vi "Find API Tester Path.vi"(8 "error in":errorcluster, 11 "DQMH Library Ref":refnum<vi>) -> (0 "error out":errorcluster, 2 "Api tester found?":bool, 3 "API Tester Path":path)   [LabVIEW 2020, in "Panther Dashboard.lvlib"]
uses:
  Panther Dashboard.lvlib
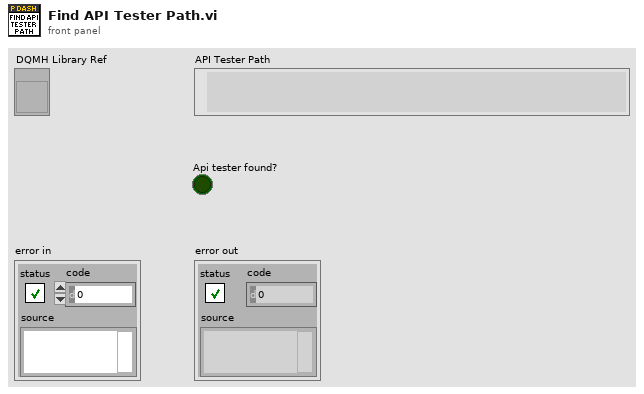
[diagram p1: front panel]
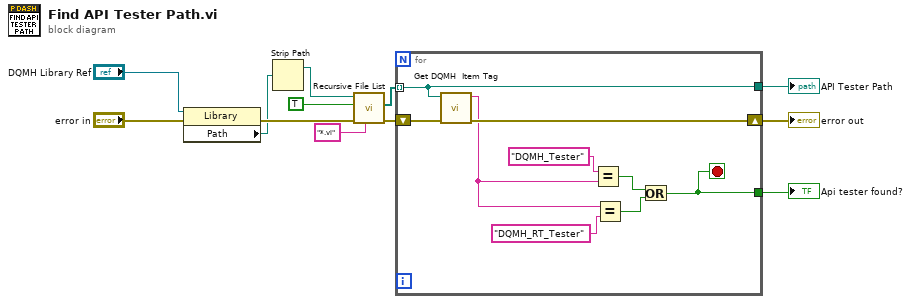
[diagram p0: block diagram]
diagram:
  n1 = property class="Library"(reference="DQMH Library Ref", error in="error in") -> (error out=w11:errorcluster, "Path"=w2:path)  [unwired: 1 out]
  n2 = Strip Path(path=w2) -> (stripped path=w3:path)  [unwired: 1 out]
  n3 = call <vilib>:"Recursive File List.vi"("pattern"="*.vi", "error in (no error)"=w11, "Treat LLBs as Folders?"=TRUE, "Folder Path"=w3) -> ("error out"=w10:errorcluster, "All Files in Dir"=w4:path[])  [unwired: 3 in, 3 out]
  n4 = for {
    tunnel: w4 -> [w19] mode=indexing
    tunnel: [w19] -> w8
    shift-right: [w20] -> w9
    shift-left: w10 -> [w21]
    tunnel: [w15] -> w6
    stop <- w15 stop-if-true
    n5 = call "Get DQMH  Item Tag.vi"("error in"=w21, "Path"=w19) -> ("error out"=w20:errorcluster, "DQMH Tag"=w13:string)  [unwired: 8 in]
    n6 = Equal?(x="DQMH_Tester" ("Tag Name"), y=w13) -> (x = y?=w17:bool)
    n7 = Equal?(x=w13, y="DQMH_RT_Tester" ("Tag Name")) -> (x = y?=w14:bool)
    n8 = Or(x=w17, y=w14) -> (x .or. y?=w15:bool)
  }
  "API Tester Path" <- w8
  "error out" <- w9
  "Api tester found?" <- w6
